vi "Module Type.vi"(11 "DAQmxDO in":refnum<class "DAQmxDO.lvclass">) -> (2 "Module Type":string)   [LabVIEW 2020, in "VolatusDAQ.lvlib" / "DAQmxDO.lvclass"]
uses:
  DAQmxDO.lvclass
  DAQmxDO.lvclass/DAQmxDO.ctl
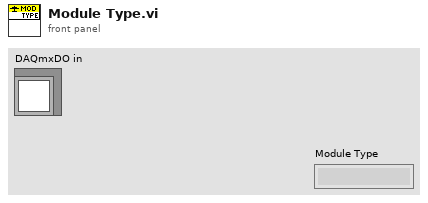
[diagram p1: front panel]
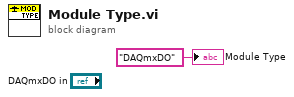
[diagram p0: block diagram]
diagram:
  "Module Type" <- "DAQmxDO" ("Module Type")
